vi "Reading DI NAME.vi"(8 "error in (no error)":errorcluster caption="错误输入（无错误）") -> (0 "error out":errorcluster caption="错误输出", 3 "Input Registers":u16[](array[numeric]))   [LabVIEW 2010]
uses:
  Source Code/SubVIs/NI Modbus.llb/MB Serial Master Query Read Input Registers (poly).vi
  SubVIs/Controller Communication.llb/F4 Controller handle Global Function Enum.ctl
panel:
  out "字符串":string
  out "*(类型 *) &x":string
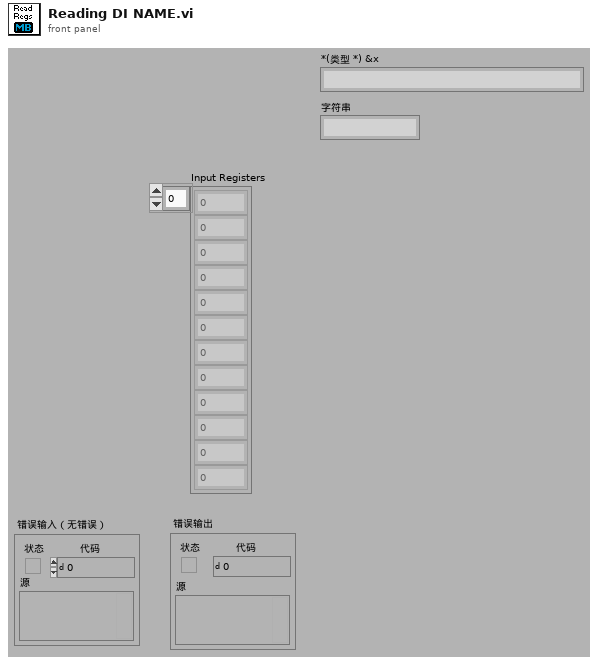
[diagram p1: front panel]
types:
  T1 = cluster{"Mode":enum16{"RTU", "ASCII"}, "Slave Address":u8}
  T2 = typedef "F4 Controller handle Global Function Enum.ctl" = enum16{"保存信息", "读取信息", "读取控制器列表", "选择控制器", "初始化"}
  T3 = typedef "F4 Controller handle.ctl" = cluster{"F4Ctrller Name":string, "Ctrller Address":i32, "VISA handle":refnum<visa-resource-name>}
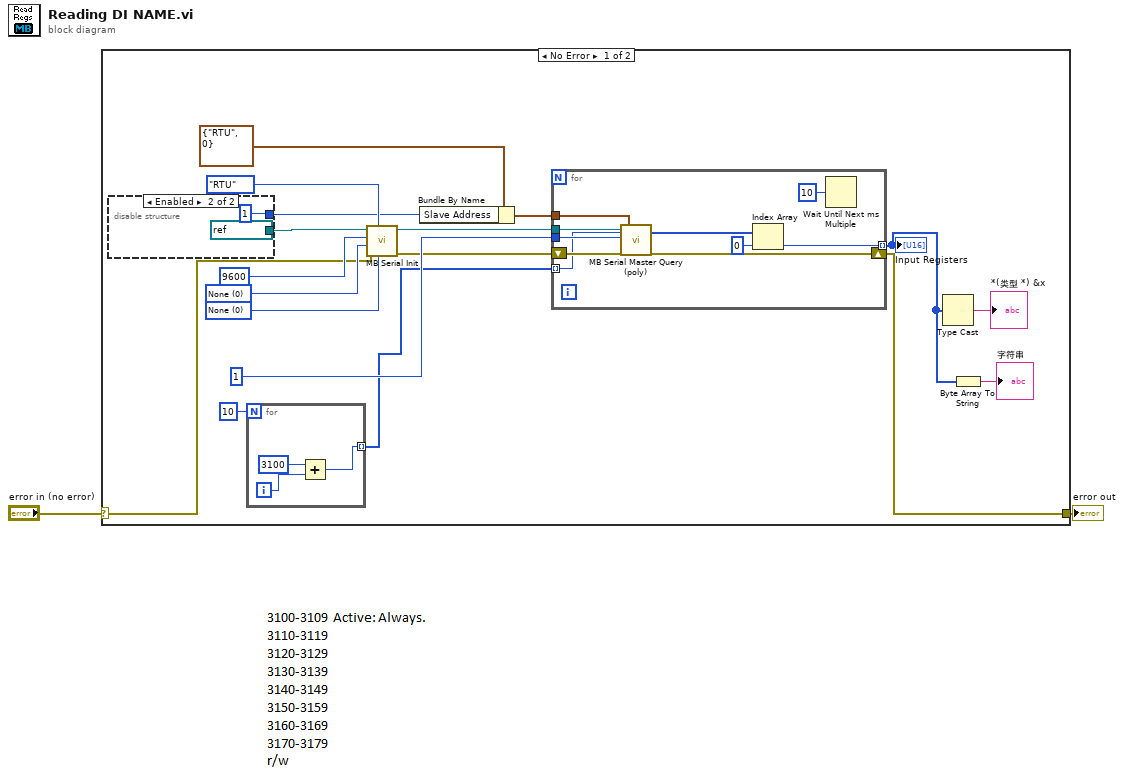
[diagram p0: block diagram]
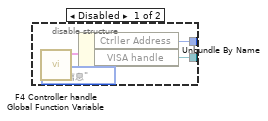
[diagram p2: hidden frame]
diagram:
  n1 = case shown="No Error" "error in (no error)" {
    selector: "error in (no error)" -> [w9 w40]
    tunnel: [w8 w40] -> w1
    frame No Error {
      w18 = u16 0 items=["None", "XON/XOFF", "RTS/CTS", "XON/XOFF & RTS/CTS", "DTR/DSR", "XON/XOFF & DTR/DSR"] ("Flow Control")
      w17 = u16 0 items=["None", "Odd", "Even", "Mark", "Space"] ("Parity")
      n2 = disable-structure shown="Enabled" {
        disable-tunnel: [w27 refnum<visa-resource-name> "COM1" ("VISA resource name")] -> w14
        disable-tunnel: [w26 1 ("Ctrller Address")] -> w13
        frame Disabled {
          n3 = call "F4 Controller handle Global Function Variable.vi"("F4 Controller handle Global Function Enum"=F4_Controller_handle_Global_Function_Enum."读取信息") -> ("控制器信息"=w25:T3)  [unwired: 7 in, 3 out]
          n4 = Unbundle By Name(w25) -> ("Ctrller Address"=w26:i32, "VISA handle"=w27:refnum<visa-resource-name>)
        }
        frame Enabled {
        }
      }
      n5 = for {
        N: 10 -> [_]
        tunnel: [w21] -> w6 mode=indexing
        i -> [w23]
        n6 = Add(x=3100, y=w23) -> (x+y=w21:i32)
      }
      n7 = call "MB Serial Init.vi"("Flow Control"=w18, "Mode"=enum16{"RTU", "ASCII"}."RTU", "error in (no error)"=w9, "Parity"=w17, "Baud Rate"=u32 9600, "VISA resource name"=w14) -> ("error out"=w19:errorcluster, "VISA resource name out"=w10:refnum<visa-resource-name>)  [unwired: 4 in]
      n8 = Bundle By Name(cluster=T1 {"Mode"=enum."RTU", "Slave Address"=0} ("Serial Parameters"), "Slave Address"=w13) -> (w12:T1)
      n9 = for {
        tunnel: u16 1 ("Quantity") -> [w37]
        tunnel: w12 -> [w35]
        tunnel: w10 -> [w34]
        tunnel: w6 -> [w32] mode=indexing
        tunnel: [w30] -> w4 mode=indexing
        shift-right: [w33] -> w8
        shift-left: w19 -> [w36]
        n10 = call-poly "MB Serial Master Query (poly).vi"("VISA resource name"=w34, "Starting Address"=w32, "Quantity"=w37, "error in"=w36, "Serial Parameters"=w35) -> ("Input Registers"=w38:u16[], "error out"=w33:errorcluster)  [unwired: 11 in, 2 out]
        n11 = Index Array(array=w38, index=0 ("索引")) -> (element=w30:u16)
        n12 = Wait Until Next ms Multiple(millisecond multiple=u32 10 ("毫秒倍数")) -> ()  [unwired: 1 out]
      }
      "Input Registers" <- w4
      n13 = Type Cast(x=w4) -> (*(type *) &x=→"*(类型 *) &x":string)  [unwired: 1 in]
      n14 = Byte Array To String(unsigned byte array=w4) -> (string=→"字符串":string)
    }
    frame Error {
    }
  }
  "error out" <- w1
